vi "PiCamera.vi"() -> ()   [LabVIEW 2019]
uses:
  <vilib>/picture/picture.llb/imagedata.ctl
  <vilib>/httpClient/POSTBuffer.vi
  <vilib>/Platform/browser.llb/Open URL in Default Browser (string).vi
  <vilib>/httpClient/LabVIEWHTTPClient.lvlib
panel:
  out "last image":T1
  in  "Save":bool
  out "class":string
  in  "Watson":bool
  in  "SDCard":bool
  in  "SSH":bool
  in  "ping":bool
  in  "Quit":bool
  in  "Snap":bool
  in  "Webpage":bool
  in  "Grab":bool
  out "new picture":picture
  in  "url":string="http://172.16.140.244"
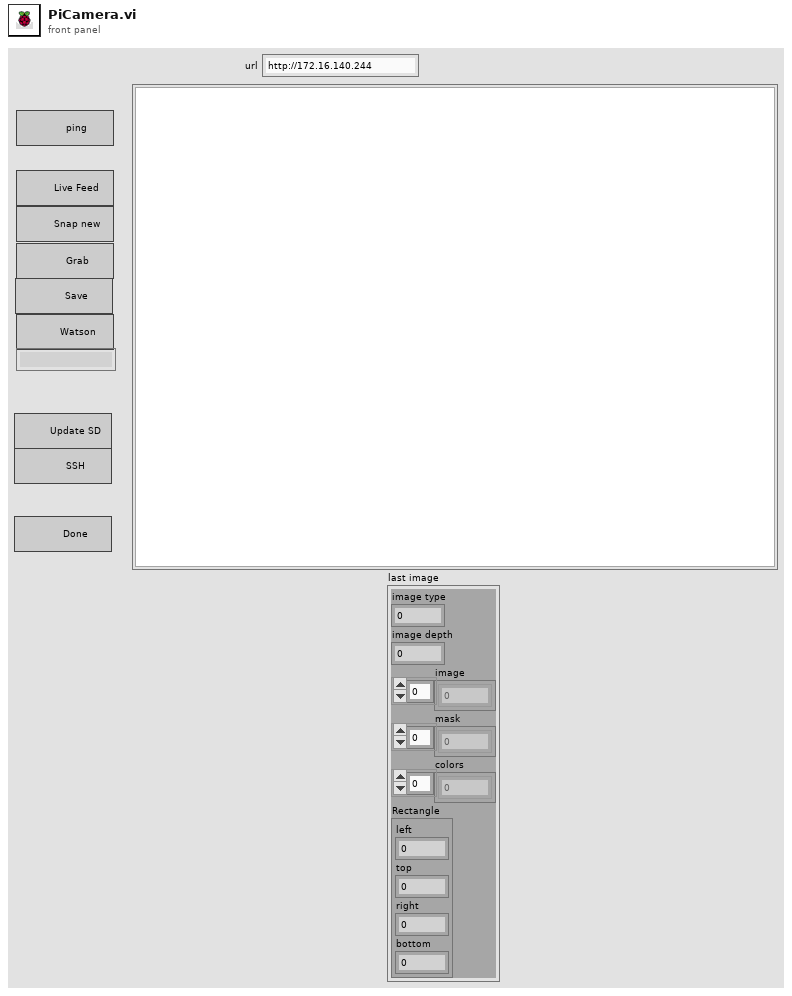
[diagram p1: front panel]
types:
  T1 = typedef "imagedata.ctl" = cluster{"image type":i32, "image depth":i32, "image":u8[], "mask":u8[], "colors":u32[], "Rectangle":cluster{"left":i16, "top":i16, "right":i16, "bottom":i16}}
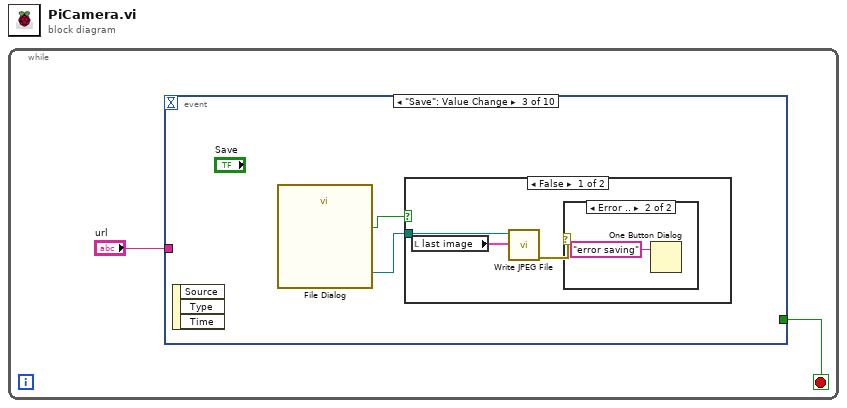
[diagram p0: block diagram]
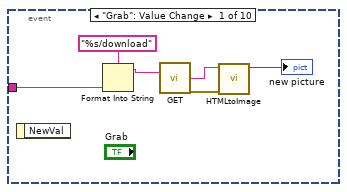
[diagram p2: hidden frame]
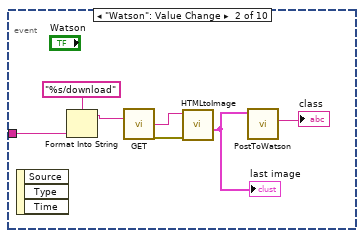
[diagram p3: hidden frame]
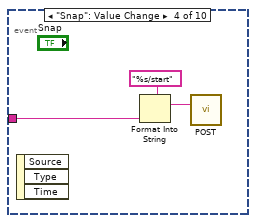
[diagram p6: hidden frame]
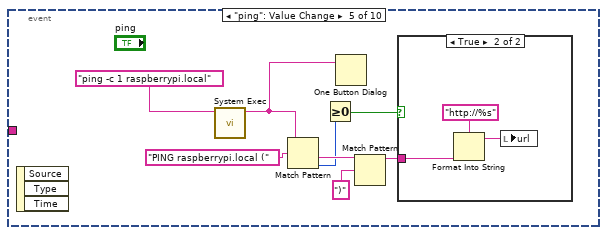
[diagram p7: hidden frame]
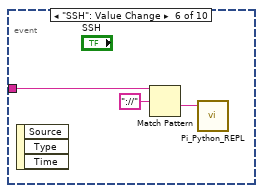
[diagram p9: hidden frame]
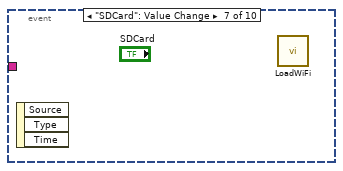
[diagram p10: hidden frame]
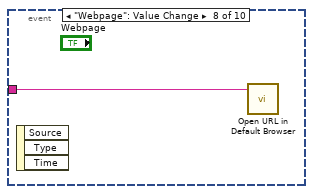
[diagram p11: hidden frame]
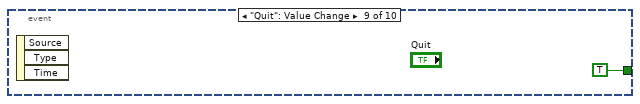
[diagram p12: hidden frame]
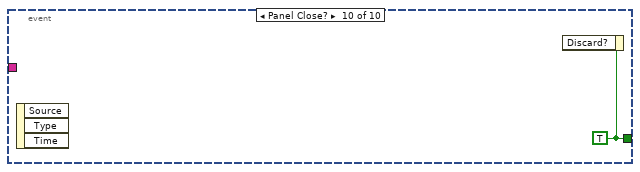
[diagram p13: hidden frame]
diagram:
  n1 = while {
    stop <- w2 stop-if-true
    n2 = event shown="[2] \"Save\": Value Change" {
      selector: _ -> [_ _ _ _ _ _ _ _ _ _]
      dyn-events: _ -> [_ _ _ _ _ _ _ _ _ _]
      timeout: _ -> [_ _ _ _ _ _ _ _ _ _]
      tunnel: "url" -> [w3 w11 _ w22 _ w38 _ w39 _ _]
      tunnel: [_ _ _ _ _ _ _ _ TRUE w41] -> w2
      event "Grab": Value Change {
        n3 = event-data() -> ()  [unwired: 1 in, 1 out]
        n4 = Format Into String(format string="%s/download" ("url"), w3) -> (resulting string=w4:string)  [unwired: 2 in, 1 out]
        n5 = call <vilib>:"GET.vi"("url"=w4) -> ("body"=w7:string, "error out"=w6:errorcluster)  [unwired: 11 in, 2 out]
        n6 = call "HTMLtoImage.vi"("error in (no error)"=w6, "body"=w7) -> ("new picture"=→"new picture":picture)  [unwired: 8 in, 1 out]
      }
      event "Watson": Value Change {
        n7 = event-data() -> ()  [unwired: 1 in, 3 out]
        n8 = Format Into String(format string="%s/download" ("url"), w11) -> (resulting string=w12:string)  [unwired: 2 in, 1 out]
        n9 = call <vilib>:"GET.vi"("url"=w12) -> ("body"=w15:string, "error out"=w14:errorcluster)  [unwired: 11 in, 2 out]
        n10 = call "HTMLtoImage.vi"("error in (no error)"=w14, "body"=w15) -> ("image data"=w10:T1)  [unwired: 8 in, 1 out]
        "last image" <- w10
        n11 = call "PostToWatson.vi"("image in"=w10) -> ("class"=→"class":string)  [unwired: 6 in, 4 out]
      }
      event "Save": Value Change {
        n12 = event-data() -> ()  [unwired: 1 in, 3 out]
        n13 = call "File Dialog"() -> ("selected path"=w17:path, "cancelled"=w16:bool)  [unwired: 12 in, 2 out]
        n14 = case shown="False" w16 {
          tunnel: w17 -> [w19 _]
          frame False {
            n15 = local read "last image"() -> (w20:T1)
            n16 = call <vilib>:"Write JPEG File.vi"("image data"=w20, "path to JPEG file"=w19) -> ("error out"=w18:errorcluster)  [unwired: 8 in, 1 out]
            n17 = case shown="Error .." w18 {
              frame No Error {
              }
              frame Error {
                n18 = One Button Dialog(message="error saving") -> ()  [unwired: 1 in, 1 out]
              }
            }
          }
          frame True {
          }
        }
      }
      event "Snap": Value Change {
        n19 = event-data() -> ()  [unwired: 1 in, 3 out]
        n20 = Format Into String(format string="%s/start" ("url"), w22) -> (resulting string=w24:string)  [unwired: 2 in, 1 out]
        n21 = call-poly <vilib>:"POST.vi"("url"=w24) -> ()  [unwired: 11 in, 4 out]
      }
      event "ping": Value Change {
        n22 = event-data() -> ()  [unwired: 1 in, 3 out]
        n23 = call <vilib>:"System Exec.vi"("command line"="ping -c 1 raspberrypi.local" ("url")) -> ("standard output"=w25:string)  [unwired: 7 in, 3 out]
        n24 = Match Pattern(string=w25, regular expression="PING raspberrypi.local (") -> (after substring=w31:string, offset past match=w29:i32)  [unwired: 1 in, 2 out]
        n25 = Greater Or Equal To 0?(x=w29) -> (x >= 0?=w28:bool)
        n26 = One Button Dialog(message=w25) -> ()  [unwired: 1 in, 1 out]
        n27 = Match Pattern(string=w31, regular expression=")") -> (before substring=w27:string)  [unwired: 1 in, 3 out]
        n28 = case shown="True" w28 {
          tunnel: w27 -> [_ w35]
          frame False {
          }
          frame True {
            n29 = Format Into String(format string="http://%s" ("url"), w35) -> (resulting string=w33:string)  [unwired: 2 in, 1 out]
            n30 = local write "url"(w33) -> ()
          }
        }
      }
      event "SSH": Value Change {
        n31 = event-data() -> ()  [unwired: 1 in, 3 out]
        n32 = Match Pattern(string=w38, regular expression="://") -> (after substring=w36:string)  [unwired: 1 in, 3 out]
        n33 = call "Pi_Python_REPL.vi"("Pi IP Address"=w36) -> ()  [unwired: 11 in]
      }
      event "SDCard": Value Change {
        n34 = event-data() -> ()  [unwired: 1 in, 3 out]
        n35 = call "LoadWiFi.vi"() -> ()  [unwired: 12 in]
      }
      event "Webpage": Value Change {
        n36 = event-data() -> ()  [unwired: 1 in, 3 out]
        n37 = call-poly <vilib>:"Open URL in Default Browser.vi"("URL"=w39) -> ()  [unwired: 5 in, 2 out]
      }
      event "Quit": Value Change {
        n38 = event-data() -> ()  [unwired: 1 in, 3 out]
      }
      event Panel Close? {
        w41 = TRUE
        n39 = event-data() -> ()  [unwired: 1 in, 3 out]
        n40 = event-data("Discard?"=w41) -> ()  [unwired: 1 in, 1 out]
      }
    }
  }
